vi "開啟圖片(2D).vi"(0 "ImageNameArray":string[](array[string])=["Source"], 5 "影像數量":i32=1, 11 "error In":errorcluster) -> (3 "ImagePath":path[](array[path]), 4 "Image2DArray":T1[][](array[typedef]), 6 "ImageNameNumber":i32, 8 "ImagePathNumber":i32, 10 "ImageOutNameArray":string[](array[string]), 15 "error out":errorcluster)   [LabVIEW 2015]
uses:
  <vilib>/vision/Image Controls.llb/IMAQ Image.ctl
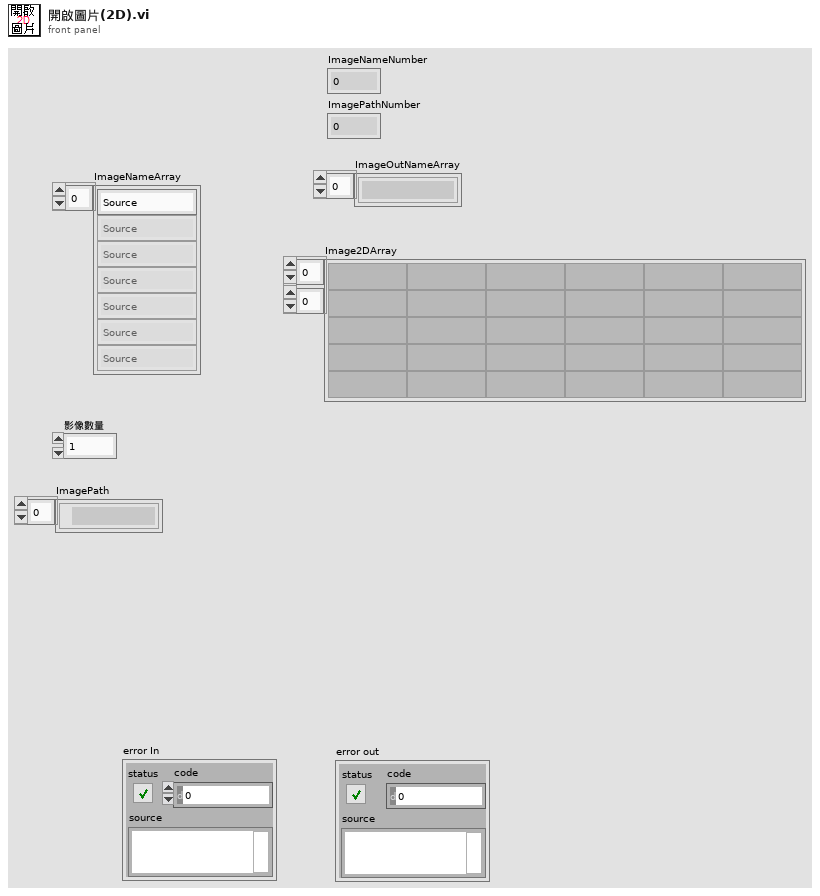
[diagram p1: front panel]
types:
  T1 = typedef "IMAQ Image.ctl" = refnum<image>
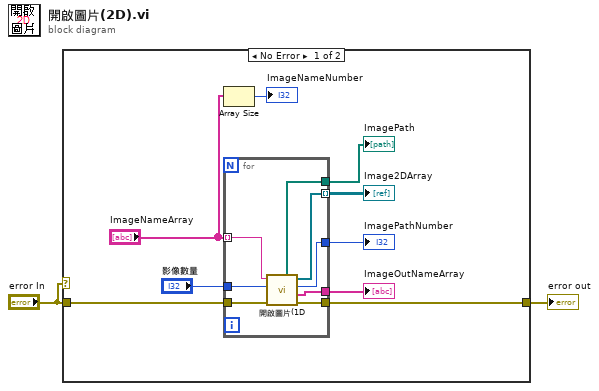
[diagram p0: block diagram]
diagram:
  n1 = case shown="No Error" "error In" {
    tunnel: [w10 w20] -> w2
    tunnel: "error In" -> [w11 w20]
    frame No Error {
      n2 = Array Size(array="ImageNameArray") -> (size(s)=→"ImageNameNumber":i32)
      n3 = for {
        tunnel: "ImageNameArray" -> [w19] mode=indexing
        tunnel: w11 -> [w17]
        tunnel: [w15] -> w10
        tunnel: "影像數量" -> [w18]
        tunnel: [w16] -> w6
        tunnel: [w14] -> w5
        tunnel: [w13] -> w4
        tunnel: [w12] -> w3 mode=indexing
        n4 = call "開啟圖片(1D.vi"("error In"=w17, "影像數量"=w18, "Image Name"=w19) -> ("error out"=w15:errorcluster, "ImageOutNameArray"=w13:string[], "ImagePathNumber"=w14:i32, "Image1DArray"=w12:T1[], "ImagePath"=w16:path[])  [unwired: 4 in]
      }
      "Image2DArray" <- w3
      "ImagePathNumber" <- w5
      "ImageOutNameArray" <- w4
      "ImagePath" <- w6
    }
    frame Error {
    }
  }
  "error out" <- w2
